vi "Plot.vi"(8 "error in (no error)":errorcluster, 11 "Spectrum Recorder in":refnum<class "Spectrum Recorder too.lvclass">) -> (0 "error out":errorcluster, 3 "Spectrum Recorder out":refnum<class "Spectrum Recorder too.lvclass">)   [LabVIEW 2019, in "Spectrum Recorder too.lvclass"]
uses:
  Spectrum Recorder too.lvclass
  C:/GitHub/LabActor/Template Module/Template Module.lvclass
  Template Module/Template Module.lvclass/Template Module.ctl
  Spectrum Recorder too.lvclass/Spectrum Recorder too.ctl
  Template Module/Read Logger.vi
  Loggers/Logger/Logger.lvclass
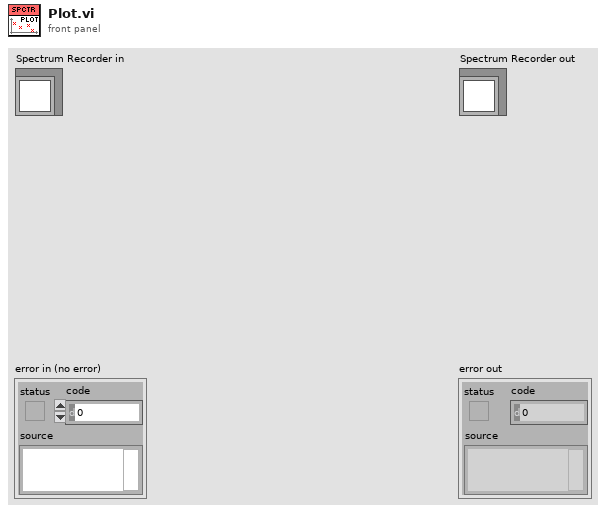
[diagram p1: front panel]
types:
  T1 = enum16{"open", "open or create", "create or replace", "create", "open (read-only)"}
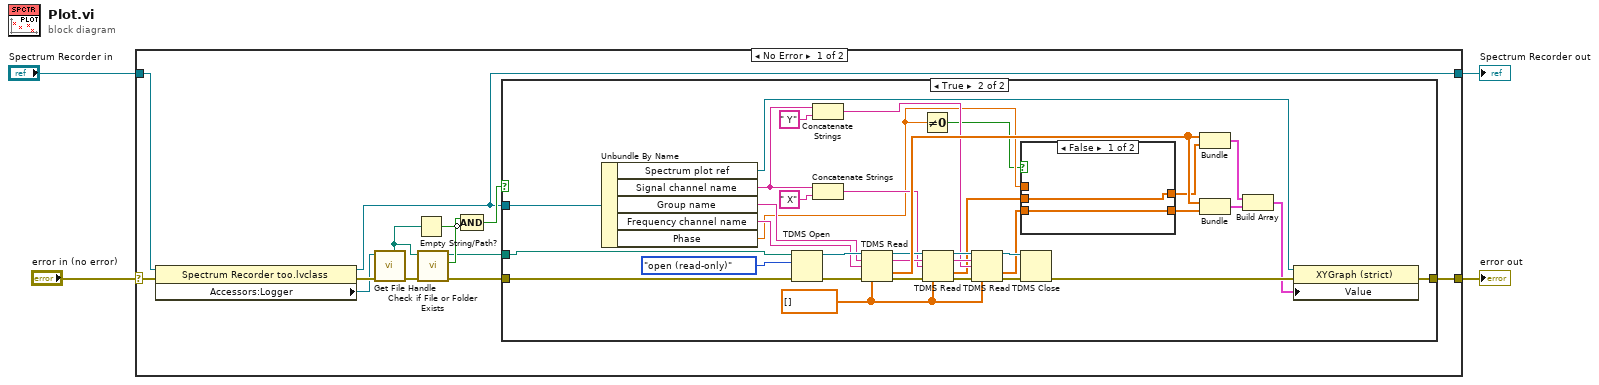
[diagram p0: block diagram]
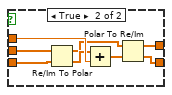
[diagram p3: hidden frame]
diagram:
  n1 = case shown="No Error" "error in (no error)" {
    selector: "error in (no error)" -> [w8 w65]
    tunnel: [w12 w65] -> w3
    tunnel: [w5 w64] -> w1
    tunnel: "Spectrum Recorder in" -> [w9 w64]
    frame No Error {
      n2 = property class="Spectrum Recorder too.lvclass"(reference=w9, error in=w8) -> (reference out=w5:refnum<class "Spectrum Recorder too.lvclass">, error out=w11:errorcluster, "Accessors:Logger"=w10:refnum<class "Logger.lvclass">)
      n3 = call-dynamic "Get File Handle.vi"("error in (no error)"=w11, "Logger in"=w10) -> ("error out"=w7:errorcluster, "Data File  Path"=w6:path)  [unwired: 5 in, 3 out]
      n4 = Empty String/Path?(string/path=w6) -> (empty?=w16:bool)
      n5 = call <vilib>:"Check if File or Folder Exists.vi"("error in (no error)"=w7, "path"=w6) -> ("error out"=w13:errorcluster, "file or folder exists?"=w17:bool, "dup path"=w14:path)  [unwired: 7 in]
      n6 = Compound Arithmetic op=AND(w17, invert w16) -> (w15:bool)
      n7 = case shown="True" w15 {
        tunnel: w14 -> [_ w51]
        tunnel: w13 -> [w18 w50]
        tunnel: w5 -> [_ w48]
        tunnel: [w18 w44] -> w12
        frame False {
        }
        frame True {
          w27 = dbl[] []
          n8 = Unbundle By Name(w48) -> ("Spectrum plot ref"=w43:refnum<vi>, "Signal channel name"=w24:string, "Group name"=w47:string, "Frequency channel name"=w46:string, "Phase"=w20:dbl)
          n9 = TDMS Open(8:w50, 10:T1."open (read-only)" ("operation (0:open)"), 11:w51) -> (0:w52:errorcluster, 3:w53:refnum<k34>)  [unwired: 4 in]
          n10 = Concatenate Strings(w24, " Y" ("string")) -> (w23:string)
          n11 = Concatenate Strings(w24, " X" ("string")) -> (w25:string)
          n12 = TDMS Read(0:w53, 5:w47, 7:w46, 11:w52, 12:w27) -> (4:w38:refnum<k34>, 6:w36:string, 10:w39:dbl[], 15:w37:errorcluster)  [unwired: 3 in, 2 out]
          n13 = Not Equal To 0?(x=w20) -> (x != 0?=w19:bool)
          n14 = TDMS Read(0:w38, 5:w36, 7:w25, 11:w37, 12:w27) -> (4:w29:refnum<k34>, 6:w26:string, 10:w22:dbl[], 15:w31:errorcluster)  [unwired: 3 in, 2 out]
          n15 = TDMS Read(0:w29, 5:w26, 7:w23, 11:w31, 12:w27) -> (4:w28:refnum<k34>, 10:w21:dbl[], 15:w30:errorcluster)  [unwired: 3 in, 3 out]
          n16 = case shown="False" w19 {
            tunnel: w20 -> [_ w62]
            tunnel: [w55 w61] -> w35
            tunnel: [w54 w60] -> w34
            tunnel: w22 -> [w55 w59]
            tunnel: w21 -> [w54 w58]
            frame False {
            }
            frame True {
              n17 = Re/Im To Polar(2:w58, 3:w59) -> (0:w57:dbl[], 1:w56:dbl[])
              n18 = Add(x=w57, y=w62) -> (x+y=w63:dbl[])
              n19 = Polar To Re/Im(2:w63, 3:w56) -> (0:w60:dbl[], 1:w61:dbl[])
            }
          }
          n20 = TDMS Close(8:w30, 11:w28) -> (0:w45:errorcluster)  [unwired: 1 out]
          n21 = Bundle(w39, w35) -> (w42:cluster{dbl[], dbl[]})  [unwired: 1 in]
          n22 = Bundle(w39, w34) -> (w41:cluster{dbl[], dbl[]})  [unwired: 1 in]
          n23 = Build Array(w42, w41) -> (w40:cluster{dbl[], dbl[]}[])
          n24 = property class="XYGraph (strict)"(reference=w43, error in=w45, "Value"=w40) -> (error out=w44:errorcluster)  [unwired: 1 out]
        }
      }
    }
    frame Error {
    }
  }
  "error out" <- w3
  "Spectrum Recorder out" <- w1
